vi "[PC]Log_GetLogFileName.vi"() -> (3 "String":string)   [LabVIEW 2018]
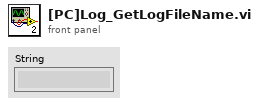
[diagram p1: front panel]
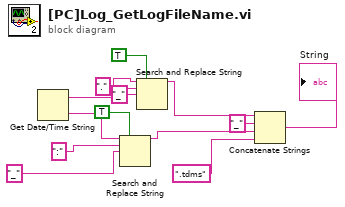
[diagram p0: block diagram]
diagram:
  n1 = Get Date/Time String() -> (date string=w3:string, time string=w6:string)  [unwired: 3 in]
  n2 = Search and Replace String(replace all?=TRUE ("replace all? (F)"), input string=w6, search string=":" ("input string"), replace string="_" ("search string")) -> (result string=w7:string)  [unwired: 4 in, 3 out]
  n3 = Search and Replace String(replace all?=TRUE ("replace all? (F)"), input string=w3, search string="." ("substring (\"\")"), replace string="_" ("replace string (\"\")")) -> (result string=w12:string)  [unwired: 4 in, 3 out]
  n4 = Concatenate Strings(w12, "_" ("string"), w7, ".tdms") -> (→"String":string)
